vi "ParseCli.vi"(8 "error in (no error)":errorcluster, 10 "Cli":string, 11 "Ping in":refnum<class "Ping.lvclass">) -> (0 "error out":errorcluster, 3 "Ping out":refnum<class "Ping.lvclass">)   [LabVIEW 2022 SP3, in "Cli.lvlib" / "Ping.lvclass"]
uses:
  Ping.lvclass
  Ping.lvclass/Ping.ctl
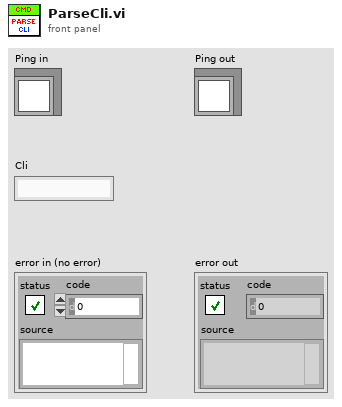
[diagram p1: front panel]
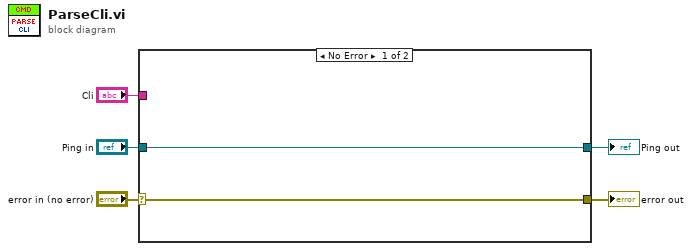
[diagram p0: block diagram]
diagram:
  n1 = case shown="No Error" "error in (no error)" {
    selector: "error in (no error)" -> [w6 w9]
    tunnel: [w6 w9] -> w5
    tunnel: [w7 w8] -> w4
    tunnel: "Cli" -> [_ _]
    tunnel: "Ping in" -> [w7 w8]
    frame No Error {
    }
    frame Error {
    }
  }
  "error out" <- w5
  "Ping out" <- w4
